vi "Create Trigger Model Dynamic Delay Block.vi"(8 "error in (no error)":errorcluster, 9 "User Delay":u16(ring)=6 items=["Measure 1"=6, "Measure 2"=7, "Measure 3 "=8, "Measure 4"=9, "Measure 5"=10], 10 "Block Number (1)":i32=1 min=1 format="%#.6g", 11 "VISA resource name":refnum<visa-resource-name>) -> (0 "error out":errorcluster, 3 "VISA resource name out":refnum<visa-resource-name>)   [LabVIEW 2016, in "Keithley DMM7510.lvlib"]
doc: "This VI adds a delay to the execution of the trigger model."
uses:
  Keithley DMM7510.lvlib
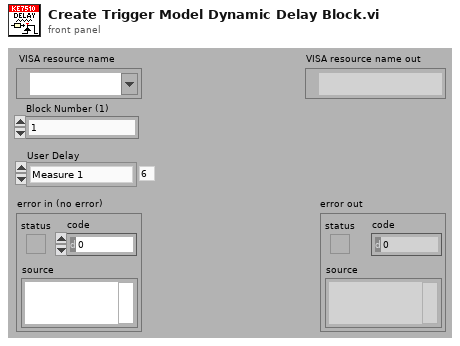
[diagram p1: front panel]
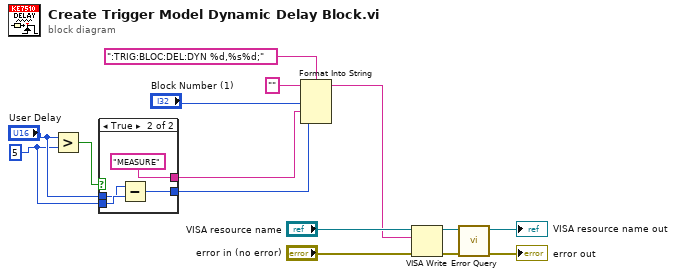
[diagram p0: block diagram]
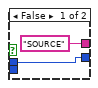
[diagram p2: hidden frame]
diagram:
  w2 = u16 5 ("y")
  n1 = Greater?(x="User Delay", y=w2) -> (0:w5:bool)
  n2 = case shown="True" w5 {
    tunnel: ["SOURCE" ("format string") "MEASURE" ("format string")] -> w4
    tunnel: "User Delay" -> [w16 w19]
    tunnel: w2 -> [_ w20]
    tunnel: [w16 w18] -> w1
    frame False {
    }
    frame True {
      n3 = Subtract(x=w19, y=w20) -> (x-y=w18:u16)
    }
  }
  n4 = Format Into String(format string=":TRIG:BLOC:DEL:DYN %d,%s%d;", initial string="", "Block Number (1)", w4, w1) -> (resulting string=w7:string)  [unwired: 1 in, 1 out]
  n5 = VISA Write(VISA resource name="VISA resource name", write buffer=w7, error in (no error)="error in (no error)") -> (VISA resource name out=w11:refnum<visa-resource-name>, error out=w10:errorcluster)  [unwired: 1 out]
  n6 = call "Error Query.vi"("error in (no error)"=w10, "VISA resource name"=w11) -> ("error out"=→"error out":errorcluster, "VISA resource name out"=→"VISA resource name out":refnum<visa-resource-name>)  [unwired: 8 out]
